vi "Autofocus_wip.vi"(0 "controller in":refnum<k24>, 1 "AbortAutoFocus":bool, 2 "ImageIn":T2, 5 "SafeMaxZ":dbl=86.0 format="%#_13g", 7 "InitialStepSize":dbl=0.1, 9 "Tolerance":dbl=0.005 format="%#_13g", 11 "error in (no error)":errorcluster, 12 "SessionIn":T1) -> (4 "controller out":refnum<k24>, 6 "Image":T2(plugin-control), 8 "N_iterations":dbl, 10 "BestZvalue":dbl, 14 "Session Out":T1, 15 "error out":errorcluster)   [LabVIEW 2019]
uses:
  C:/Users/TTUHEP/Documents/LabVIEW/Other Models/2010/Bin/Aerotech.A3200.dll
  Other Models/2010/Bin/Aerotech.A3200.dll
  <vilib>/vision/Image Controls.llb/IMAQ Image.ctl
  <vilib>/userDefined/High Color/IMAQdx.ctl
  <vilib>/Utility/error.llb/DialogType.ctl
  <vilib>/vision/NI_Vision_Development_Module.lvlib
  <vilib>/vision/driver/NI_Vision_Acquisition_Software.lvlib
panel:
  in  "Buffer Number":u32
  in  "Frames per Second Update Interval (ms)":u32=1
  in  "Minimum Display Update Interval (ms)":u32=100
  out "Images Missed":u32
  out "Processed Frames per Second":dbl
  out "Acquired Frames per Second":dbl
  out "Buffer Number Out":u32
  out "ZvsSD":string
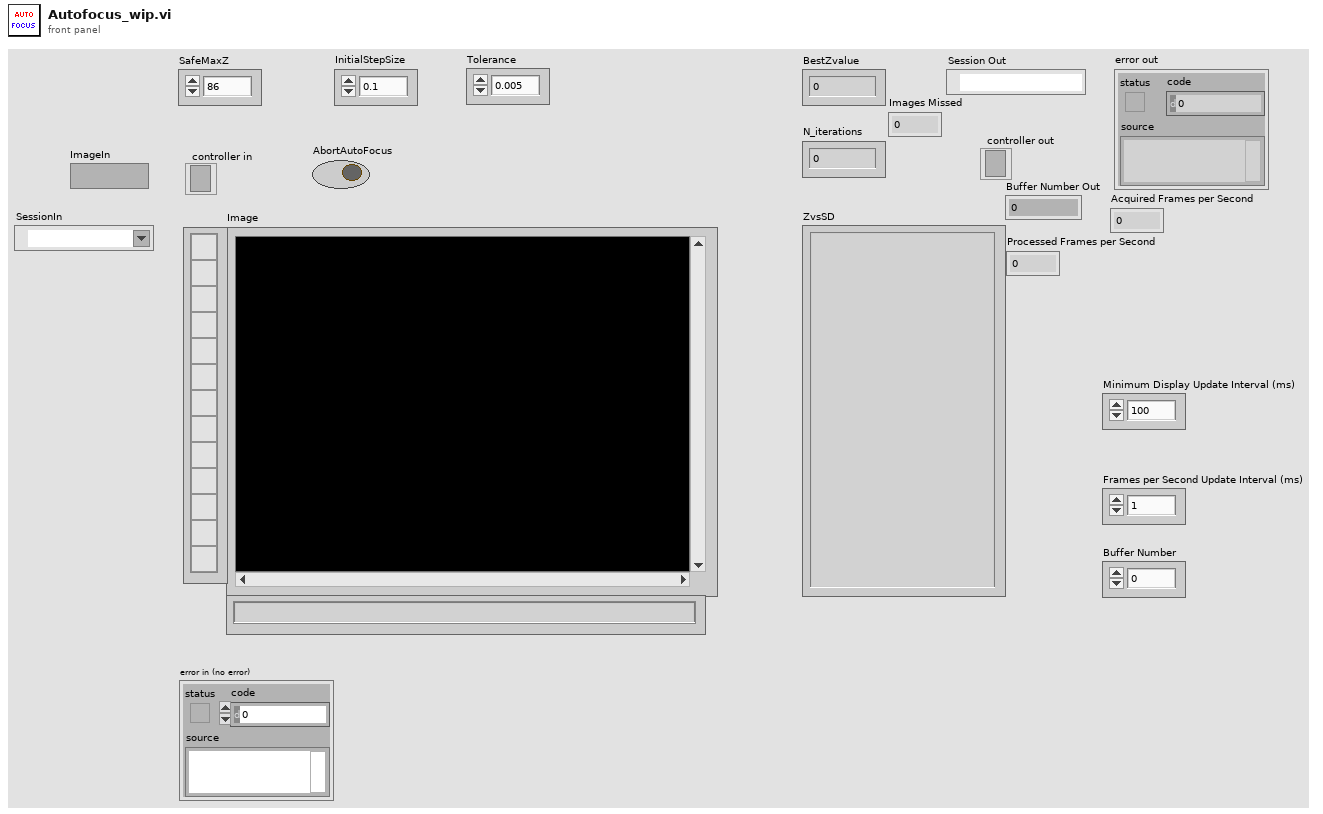
[diagram p1: front panel]
types:
  T1 = typedef "IMAQdx.ctl" = refnum<k21>
  T2 = typedef "IMAQ Image.ctl" = refnum<image>
  T3 = enum32{"Differentiation", "Gradient", "Prewitt", "Roberts", "Sigma", "Sobel"}
  T4 = typedef "Image Type" = u32
  T5 = typedef "DialogType.ctl" = u16
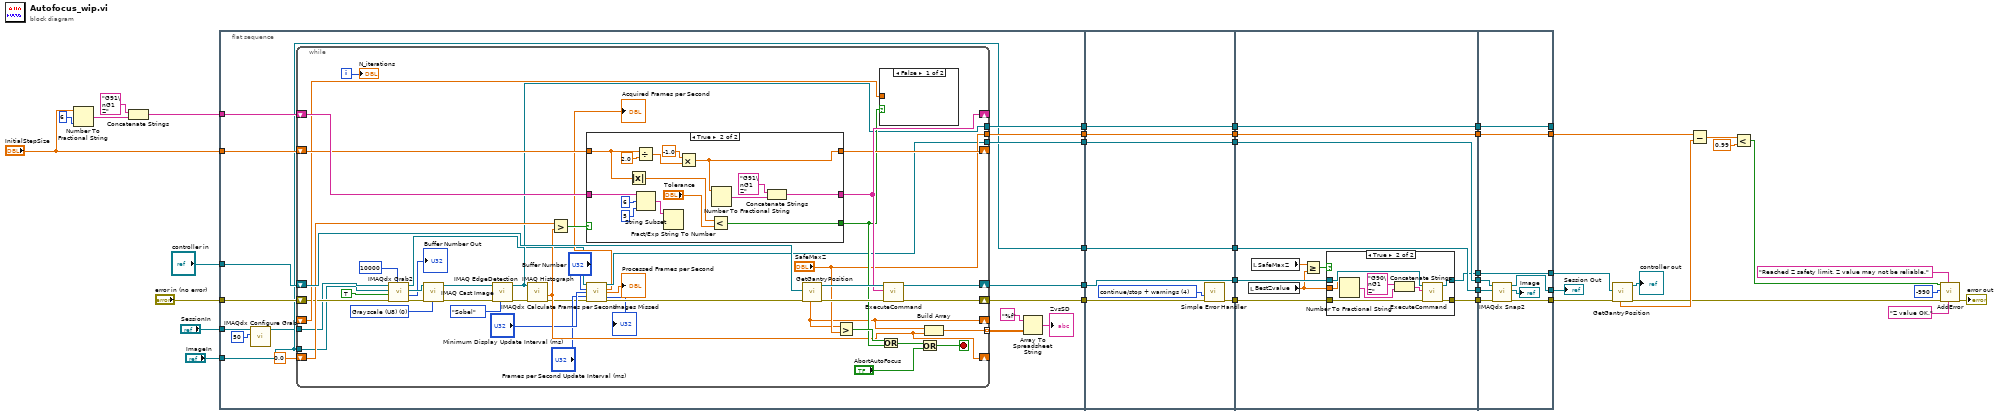
[diagram p0: block diagram]
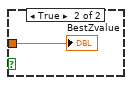
[diagram p2: hidden frame]
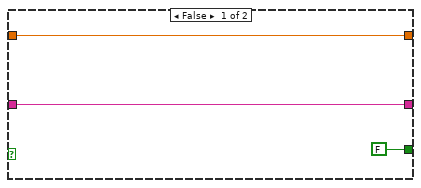
[diagram p3: hidden frame]
diagram:
  n1 = Number To Fractional String(number="InitialStepSize", precision (6)=i16 6) -> (F-format string=w37:string)  [unwired: 2 in]
  n2 = Concatenate Strings("G91\nG1 Z", w37) -> (w39:string)
  n3 = flat-sequence {
    tunnel: "controller in" -> [w58]
    tunnel: "InitialStepSize" -> [w56]
    tunnel: w39 -> [w55]
    tunnel: "error in (no error)" -> [w54]
    tunnel: [w53] -> w17
    tunnel: [w52] -> w15
    tunnel: [w51] -> w13
    tunnel: [w50] -> w11
    tunnel: [w49] -> w9
    tunnel: "SessionIn" -> [w44]
    tunnel: "ImageIn" -> [w48]
    tunnel: [w48] -> w7
    tunnel: w17 -> [w131]
    tunnel: [w131] -> w16
    tunnel: w15 -> [w130]
    tunnel: [w130] -> w14
    tunnel: w13 -> [w125]
    tunnel: [w124] -> w12
    tunnel: w11 -> [w129]
    tunnel: [w129] -> w10
    tunnel: w9 -> [w128]
    tunnel: [w128] -> w8
    tunnel: w7 -> [w127]
    tunnel: [w127] -> w6
    tunnel: w16 -> [w138]
    tunnel: [w135] -> w23
    tunnel: w14 -> [w142]
    tunnel: [w142] -> w22
    tunnel: w12 -> [w137]
    tunnel: [w136] -> w21
    tunnel: w10 -> [w141]
    tunnel: [w141] -> w20
    tunnel: w8 -> [w140]
    tunnel: [w140] -> w19
    tunnel: w6 -> [w139]
    tunnel: [w139] -> w18
    tunnel: [w159] -> _
    tunnel: [w160] -> w25
    tunnel: [w161] -> w36
    tunnel: w23 -> [w161]
    tunnel: w22 -> [w160]
    tunnel: w21 -> [w158]
    tunnel: w20 -> [w159]
    tunnel: [w157] -> w2
    tunnel: [w156] -> w1
    tunnel: w19 -> [w154]
    tunnel: w18 -> [w153]
    frame #0 {
      n4 = call <vilib>:"IMAQdx Configure Grab.vi"("Number of Buffers"=u32 50, "Session In"=w44) -> ("Session Out"=w43:T1)  [unwired: 8 in, 1 out]
      n5 = while {
        shift-right: [w96] -> w53
        shift-left: w58 -> [w100]
        shift-right: [w98] -> w51
        shift-left: w54 -> [w80]
        shift-right: [w93] -> _
        shift-left: w55 -> [w92]
        shift-right: [w72] -> _
        shift-left: 0.0 -> [w95]
        shift-right: [w89] -> _
        shift-left: w56 -> [w88]
        shift-right: [w73] -> _
        shift-left: _ -> [w87]
        tunnel: ["SafeMaxZ"] -> w52
        tunnel: [w82] -> w50
        tunnel: w48 -> [w78]
        tunnel: w43 -> [w79]
        tunnel: [w68] -> w49
        tunnel: [w74] -> w45 mode=indexing
        i -> [w84]
        stop <- w102 stop-if-true
        w85 = T4 0 items=["Grayscale (U8)", "Grayscale (I16)", "Grayscale (SGL)", "Complex (CSG)", "RGB (U32)", "HSL (U32)", "RGB (U64)", "Grayscale (U16)"] ("Image Type")
        n6 = call <vilib>:"IMAQdx Grab2.vi"("Timeout (ms)"=10000, "error in"=w80, "Wait for Next Buffer? (Yes)"=TRUE, "Image In"=w78, "Session In"=w79) -> ("error out"=w81:errorcluster, "Buffer Number Out"=→"Buffer Number Out":u32, "Image Out"=w77:T2, "Session Out"=w60:T1)  [unwired: 3 in]
        n7 = call "IMAQ Cast Image"("Image Type"=w85, "error in (no error)"=w81, "Image Src"=w77) -> ("error out"=w75:errorcluster, "Image Dst Out"=w101:T2)  [unwired: 7 in]
        n8 = call "IMAQ EdgeDetection"("Method"=T3."Sobel", "error in (no error)"=w75, "Image Src"=w101) -> ("error out"=w104:errorcluster, "Image Dst Out"=w82:T2)  [unwired: 7 in]
        n9 = call "IMAQ Histograph"("error in (no error)"=w104, "Image"=w82) -> ("error out"=w62:errorcluster, "Standard  Deviation"=w72:sgl)  [unwired: 6 in, 2 out]
        n10 = Greater?(x=w95, y=w72) -> (0:w94:bool)
        n11 = case shown="True" w94 {
          tunnel: [w108 w122] -> w93
          tunnel: w92 -> [w108 w116]
          tunnel: [FALSE w117] -> w86
          tunnel: [w106 w112] -> w89
          tunnel: w88 -> [w106 w109]
          frame False {
          }
          frame True {
            n12 = Absolute Value(x=w109) -> (abs(x)=w110:dbl)
            n13 = Divide(x=w109, y=2.0) -> (x/y=w111:dbl)
            n14 = String Subset(string=w116, offset (0)=6, length (rest)=5) -> (substring=w113:string)
            n15 = Fract/Exp String To Number(string=w113) -> ()  [unwired: 3 in, 2 out]
            n16 = Multiply(x=-1.0, y=w111) -> (x*y=w112:dbl)
            n17 = Less?(x=w110, y="Tolerance") -> (x < y?=w117:bool)
            n18 = Number To Fractional String(number=w112) -> (F-format string=w121:string)  [unwired: 3 in]
            n19 = Concatenate Strings("G91\nG1 Z", w121) -> (w122:string)
          }
        }
        n20 = call <vilib>:"IMAQdx Calculate Frames per Second.vi"("Session In"=w60, "Buffer Number"="Buffer Number", "Minimum Display Update Interval (ms)"="Minimum Display Update Interval (ms)", "Frames per Second Update Interval (ms)"="Frames per Second Update Interval (ms)", "error in (no error)"=w62) -> ("Session Out"=w68:T1, "Acquired Frames per Second"=→"Acquired Frames per Second":dbl, "Processed Frames per Second"=→"Processed Frames per Second":dbl, "Images Missed"=→"Images Missed":u32, "error out"=w61:errorcluster)  [unwired: 4 in, 2 out]
        n21 = call "GetGantryPosition.vi"("error in (no error)"=w61, "Controller In"=w100) -> ("error out"=w99:errorcluster, "controller out"=w97:refnum<k24>, "Position Z"=w73:dbl)  [unwired: 3 in, 4 out]
        n22 = Greater?(x=w73, y="SafeMaxZ") -> (0:w91:bool)
        n23 = case shown="False" w86 {
          tunnel: w87 -> [_ w105]
          frame False {
          }
          frame True {
            "BestZvalue" <- w105
          }
        }
        n24 = Or(x=w91, y=w86) -> (x .or. y?=w90:bool)
        n25 = call "ExecuteCommand.vi"("error in (no error)"=w99, "Command Code"=w93, "controller in"=w97) -> ("error out"=w98:errorcluster, "controller out"=w96:refnum<k24>)  [unwired: 6 in, 1 out]
        n26 = Or(x=w90, y="AbortAutoFocus") -> (x .or. y?=w102:bool)
        n27 = Build Array(w73, w72) -> (w74:dbl[])
        "N_iterations" <- w84
      }
      n28 = Array To Spreadsheet String(array=w45, 3:"%f" ("format string")) -> (spreadsheet string=→"ZvsSD":string)  [unwired: 1 in]
    }
    frame #1 {
      w126 = T5 4 items=["no dialog", "OK message", "continue or stop message", "OK message + warnings", "continue/stop + warnings"] ("type of dialog (OK msg:1)")
      n29 = call <vilib>:"Simple Error Handler.vi"("type of dialog (OK msg:1)"=w126, "error in (no error)"=w125) -> ("error out"=w124:errorcluster)  [unwired: 3 in, 4 out]
    }
    frame #2 {
      n30 = local read "BestZvalue"() -> (w133:dbl)
      n31 = local read "SafeMaxZ"() -> (w134:dbl)
      n32 = Greater Or Equal?(x=w134, y=w133) -> (x >= y?=w132:bool)
      n33 = case shown="True" w132 {
        tunnel: w138 -> [w144 w152]
        tunnel: w137 -> [w143 w151]
        tunnel: [w143 w147] -> w136
        tunnel: [w144 w146] -> w135
        tunnel: w133 -> [_ w145]
        frame False {
        }
        frame True {
          n34 = Number To Fractional String(number=w145) -> (F-format string=w150:string)  [unwired: 3 in]
          n35 = Concatenate Strings("G90\nG1 Z", w150) -> (w148:string)
          n36 = call "ExecuteCommand.vi"("error in (no error)"=w151, "Command Code"=w148, "controller in"=w152) -> ("error out"=w147:errorcluster, "controller out"=w146:refnum<k24>)  [unwired: 6 in, 1 out]
        }
      }
    }
    frame #3 {
      n37 = call <vilib>:"IMAQdx Snap2.vi"("error in"=w158, "Image In"=w153, "Session In"=w154) -> ("error out"=w157:errorcluster, "Image Out"=→"Image":T2, "Session Out"=w156:T1)  [unwired: 6 in]
    }
  }
  n38 = call "GetGantryPosition.vi"("error in (no error)"=w2, "Controller In"=w36) -> ("error out"=w29:errorcluster, "controller out"=→"controller out":refnum<k24>, "Position Z"=w34:dbl)  [unwired: 3 in, 4 out]
  n39 = Subtract(x=w25, y=w34) -> (x-y=w33:dbl)
  n40 = Less?(x=w33, y=0.99) -> (x < y?=w31:bool)
  n41 = call "AddError.vi"("NoErrorMessage"="Z value OK.", "ErrorMessage"="Reached Z safety limit. Z value may not be reliable.", "error in"=w29, "code"=-990, "Error?"=w31) -> ("Error out"=→"error out":errorcluster)  [unwired: 6 in]
  "Session Out" <- w1
